vi "sensors.vi"() -> ()   [LabVIEW 2019]
doc: "This global variable contains sensor readings."
panel:
  out "Retrieved_Shooter_1_Power":dbl
  out "Retrieved_Shooter_0_Power":dbl
  out "Beam_Break_Raw":i32
  out "Balls_Shot_Current":i32
  out "Retrieved_Kicker_Power":dbl
  out "Balls_Shot_Total":i32
  out "Kicker_Temp (C)":u8
  out "Kicker_Speed (rpm)":dbl
  out "Shooter_Motor_Failure":bool[](array[boolean])
  out "Retrieved_Shooter_Power":dbl
  out "Shooter_Overheat":bool[](array[boolean])
  out "Shooter_1_Temp (C)":u8
  out "Shooter_0_Temp (C)":u8
  out "Shooter_1_Speed (rpm)":dbl
  out "Shooter_0_Speed (rpm)":dbl
  out "Safe_Module_Latch_Angle (deg) [-180,180]":dbl
  out "Swerve_3_Latched_Shift_Time (ms)":u32
  out "Swerve_2_Latched_Shift_Time (ms)":u32
  out "Swerve_1_Latched_Shift_Time (ms)":u32
  out "Swerve_0_Latched_Shift_Time (ms)":u32
  out "Swerve_2_Drive_Velocity_Latched (ft/s)":dbl
  out "Swerve_3_Drive_Velocity_Latched (ft/s)":dbl
  out "Swerve_1_Drive_Velocity_Latched (ft/s)":dbl
  out "Swerve_0_Drive_Velocity_Latched (ft/s)":dbl
  out "Swerve_Shifter_Stuck":bool[](array[boolean])
  out "Swerve_Azimuth_Sensor_Fault":bool[](array[boolean])
  out "Swerve_3_Azimuth_Raw_Position (deg)":dbl
  out "Swerve_2_Azimuth_Raw_Position (deg)":dbl
  out "Swerve_1_Azimuth_Raw_Position (deg)":dbl
  out "Swerve_0_Azimuth_Raw_Position (deg)":dbl
  out "Robot_Yaw_Rate (deg/s)":dbl
  out "LimeLight_Horizontal_Offset_To_Ball (in)":dbl
  out "LimeLight_Raw_Horizontal_Offset_To_Ball (deg)":dbl
  out "LimeLight_Distance_To_Ball (in)":dbl
  out "LimeLight_Ball_Tracking_Valid":bool
  out "Swerve_Shifter_Failure":bool[](array[boolean])
  in  "Swerve_3_Actual_Shifter_State":T1(ring)
  in  "Swerve_2_Actual_Shifter_State":T1(ring)
  in  "Swerve_1_Actual_Shifter_State":T1(ring)
  in  "Swerve_0_Actual_Shifter_State":T1(ring)
  out "Swerve_Ground_Speed (ft/s)":dbl
  out "CAN_Bus_Fault":bool
  out "Pose_Loop_Time (ms)":u32
  out "LIDAR_Distance_To_Target (in)":dbl
  out "Fused_Heading_To_Target (deg)":dbl
  out "LIDAR_Range_Valid":bool
  out "LimeLight_Range_Valid":bool
  out "LimeLight_PnP_Valid":bool
  out "Control_Latency_Alarm":bool
  out "Battery_Critical":bool
  out "Electrical_Fault":bool
  out "Time_Since_Pose_Update (ms)":u32
  out "Set_Robot_Pos":bool
  out "Set_Robot_Y (in)":dbl
  out "Set_Robot_X (in)":dbl
  out "Fused_Heading_To_Target_Delta (deg)":dbl
  out "IMU_Failure":bool
  out "Intake_Overheat":bool
  out "Intake_Temp (C)":u8
  out "Pointed_At_Target":bool
  out "Fused_Distance_To_Target (in)":dbl
  out "Swerve_2_Drive_Velocity (ft/s)":dbl
  out "Swerve_3_Drive_Velocity (ft/s)":dbl
  out "Swerve_1_Drive_Velocity (ft/s)":dbl
  out "Swerve_0_Drive_Velocity (ft/s)":dbl
  out "Pressure_Leak":bool
  out "Swerve_Drive_Overheat":bool[](array[boolean])
  out "Swerve_Azimuth_Fault":bool[](array[boolean])
  out "Compressor_On":bool
  out "Pressure_Transducer (PSI)":dbl
  out "Control_Loop_Time (ms)":u32
  out "LimeLight_Power_Port_Valid":bool
  out "Battery_Voltage (V)":dbl
  out "Swerve_2_Drive_Temp (C)":u8
  out "Swerve_3_Drive_Temp (C)":u8
  out "Swerve_1_Drive_Temp (C)":u8
  out "Swerve_0_Drive_Temp (C)":u8
  out "Swerve_3_Azimuth_Position (deg)":dbl
  out "Swerve_2_Azimuth_Position (deg)":dbl
  out "Swerve_1_Azimuth_Position (deg)":dbl
  out "Swerve_0_Azimuth_Position (deg)":dbl
  out "Robot_H (deg)":dbl
  out "Push_Robot_H (deg)":dbl
  out "Push_Robot_Pos":bool
  out "Push_Robot_Y (in)":dbl
  out "Push_Robot_X (in)":dbl
  out "Robot_Y (in)":dbl
  out "Robot_X (in)":dbl
  # "--robot pose--"
  # "--targeting info--"
  # "--pressure management--"
  # "--power and electrical  management--"
  # "--compute resources--"
  # "--ball handling subsystem--"
  # "--drive subsystem--"
  # "--shooter subsystem--"
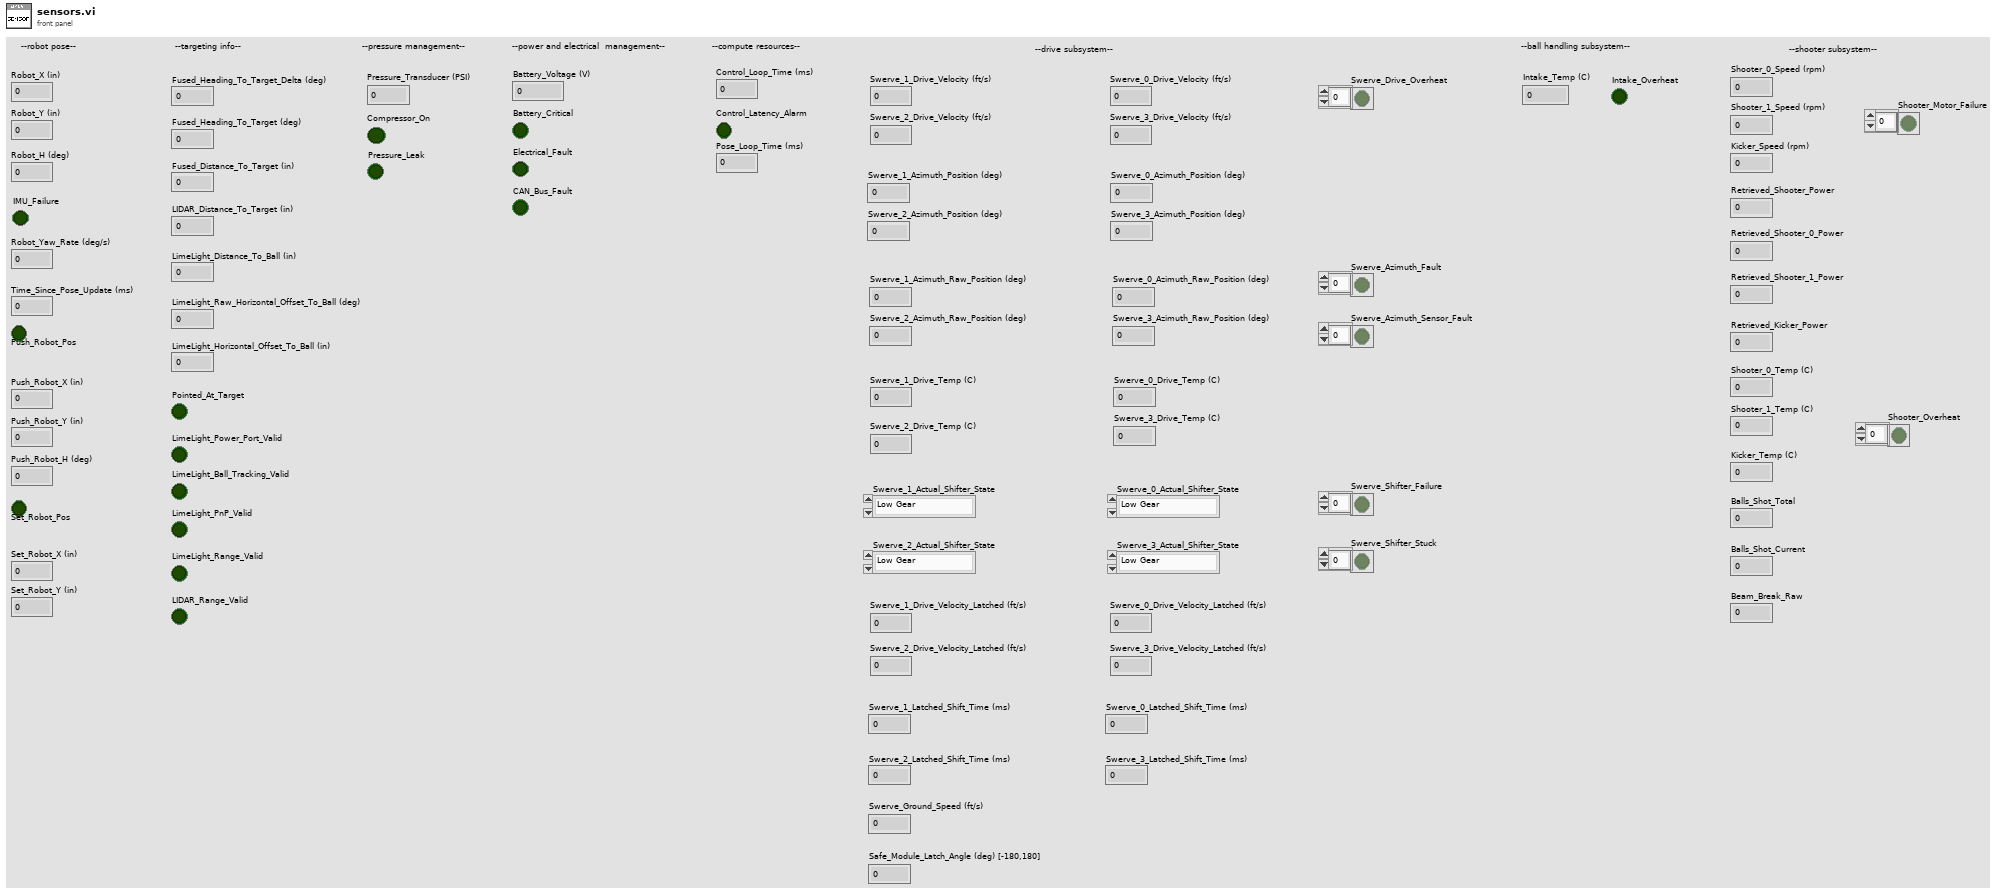
[diagram p1: front panel]
types:
  T1 = enum16{"Low Gear", "High Gear", "Transiting", "Unknown", "Force Low Gear"}
diagram:
